vi "ParseSystemDefinitionFile.vi"(8 "error in (no error)":errorcluster, 10 "VI in":refnum<vi>, 11 "System Definiton File in":path) -> (0 "error out":errorcluster, 1 "Target List out":refnum<k39>[](array[refnum]), 2 "System Definition Reference out":refnum<k39>, 3 "Absolute System Definiton File out":path)   [LabVIEW 2027, in "VeriStandTestUtilities.lvlib"]
uses:
  VeriStandTestUtilities.lvlib
  C:/NetCoreDLL/NationalInstruments.VeriStand.SystemDefinitionAPI.dll
  NetCoreDLL/NationalInstruments.VeriStand.SystemDefinitionAPI.dll
  <userlib>/_OpenG.lib/file/file.llb/Append Path to Root if Relative - Scalar__ogtk.vi
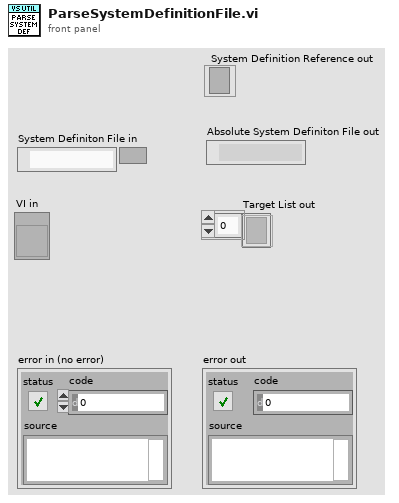
[diagram p1: front panel]
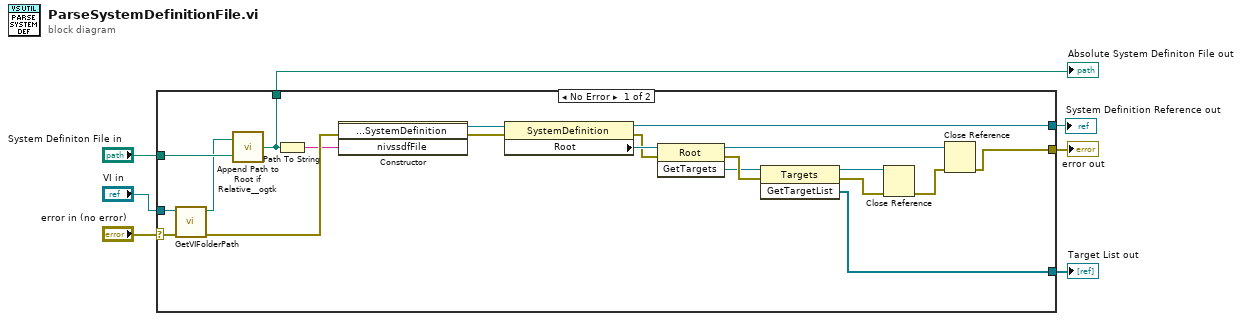
[diagram p0: block diagram]
diagram:
  n1 = case shown="No Error" "error in (no error)" {
    selector: "error in (no error)" -> [w11 w28]
    tunnel: "System Definiton File in" -> [w27 _]
    tunnel: "VI in" -> [w24 _]
    tunnel: [w23 _] -> w5
    tunnel: [w9 w28] -> w4
    tunnel: [w10 _] -> w2
    tunnel: [w8 _] -> w1
    frame No Error {
      n2 = call "GetVIFolderPath.vi"("error in (no error)"=w11, "VI Reference in"=w24) -> ("error out"=w25:errorcluster, "VI Folder Path out"=w26:path)  [unwired: 8 in]
      n3 = call-poly <userlib>:"Append Path to Root if Relative__ogtk.vi"("Absolute or Relative Path"=w27, "Root Path"=w26) -> ("Absolute or Appended Path"=w10:path)
      n4 = Path To String(path=w10) -> (string=w22:string)
      n5 = constructor class="SystemDefinition"(error in=w25, "nivssdfFile"=w22) -> (reference out=w19:refnum<k39>, error out=w20:errorcluster)  [unwired: 2 in, 2 out]
      n6 = property class="SystemDefinition"(reference=w19, error in=w20) -> (reference out=w8:refnum<k39>, error out=w17:errorcluster, "Root"=w18:refnum<k39>)
      n7 = invoke class="Root" method="GetTargets"(reference=w18, error in=w17) -> (reference out=w14:refnum<k39>, error out=w21:errorcluster, "GetTargets"=w16:refnum<k39>)  [unwired: 1 in]
      n8 = invoke class="Targets" method="GetTargetList"(reference=w16, error in=w21) -> (reference out=w13:refnum<k39>, error out=w12:errorcluster, "GetTargetList"=w23:refnum<k39>[])  [unwired: 1 in]
      n9 = Close Reference(reference=w13, error in (no error)=w12) -> (error out=w15:errorcluster)
      n10 = Close Reference(reference=w14, error in (no error)=w15) -> (error out=w9:errorcluster)
    }
    frame Error {
    }
  }
  "error out" <- w4
  "Target List out" <- w5
  "Absolute System Definiton File out" <- w2
  "System Definition Reference out" <- w1
